vi "DataAnalysis.vi"() -> ()   [LabVIEW 2012]
doc: "DWTT主界面。\n\nname: 蒋松\nEmail：jiangsong@outlook.com"
uses:
  <vilib>/Utility/miscctls.llb/LVPoint32TypeDef.ctl
  <vilib>/Utility/miscctls.llb/LVRectTypeDef.ctl
panel:
  in  "FileExplore":string[](tree)
  in  "Exit":bool
  in  "Wave Select":u16(ring) items=["力/时间", "力/位移", "能量/位移", "位移/时间", "能量/时间", "速度/时间"]
  out "落锤高度":dbl
  out "MainXY":cluster{"Time":dbl[], "Energy":dbl[]}[](graph)
  out "冲击能量的特征值（J）":T1
  out "位移的特征值（mm）":T2
  out "环境温度":dbl
  out "材料名称":dbl
  out "系统状态":string="正常"
  out "落锤质量":dbl
  out "力的特征值（N）":T3
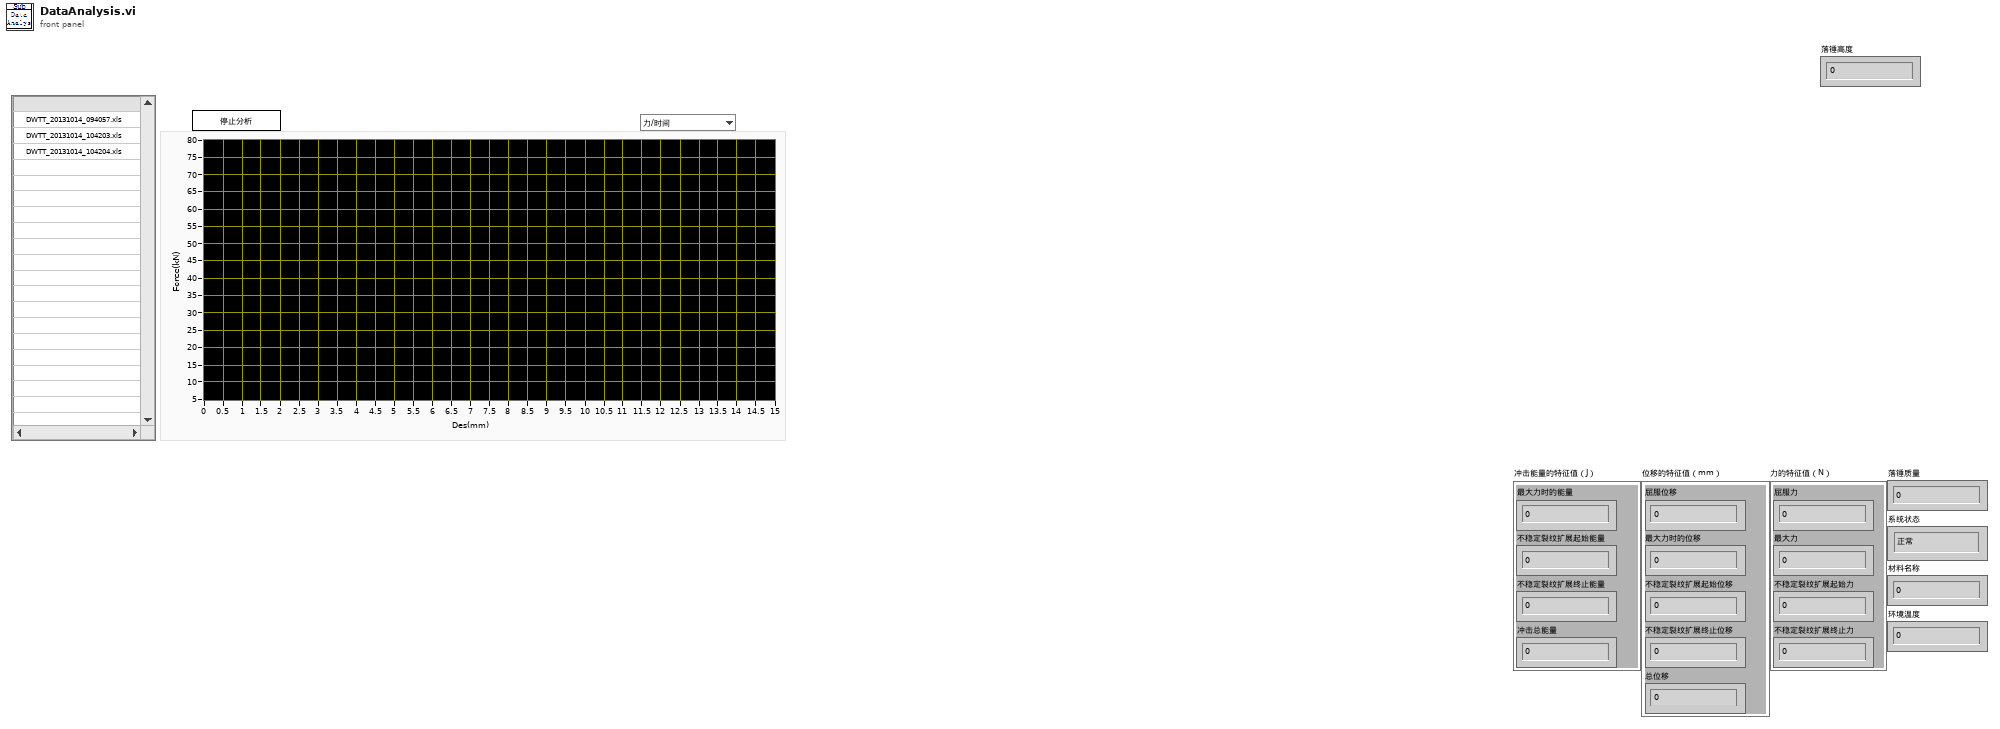
[diagram p1: front panel]
types:
  T1 = cluster{"最大力时的能量":dbl, "不稳定裂纹扩展起始能量":dbl, "不稳定裂纹扩展终止能量":dbl, "冲击总能量":dbl}
  T2 = cluster{"屈服位移":dbl, "最大力时的位移":dbl, "不稳定裂纹扩展起始位移":dbl, "不稳定裂纹扩展终止位移":dbl, "总位移":dbl}
  T3 = cluster{"屈服力":dbl, "最大力":dbl, "不稳定裂纹扩展起始力":dbl, "不稳定裂纹扩展终止力":dbl}
  T4 = enum32{"invalid app kind", "Development System", "Run Time System", "Student Edition", "Embedded LabVIEW", "Evaluation", "Custom"}
  T5 = cluster{"F/T":bool, "F/D":bool, "E/D":bool, "D/T":bool, "E/T":bool, "V/T":bool}
  T6 = typedef "LVRectTypeDef.ctl" = cluster{"Left":i16, "Top":i16, "Right":i16, "Bottom":i16}
  T7 = enum32{"Invalid", "Standard", "Closed", "Hidden", "Minimized", "Maximized"}
  T8 = cluster{"Core":cluster{"Current VI Reference":refnum<vi>, "Close Panel on Exit?":bool}, "EventPacket":cluster{"State":string, "data":variant}, "RawData":cluster{"Time":dbl[], "Force":dbl[], "Displacement":dbl[], "Velocity":dbl[], "Energy":dbl[]}[], "Tree Out":refnum<vi>, "XYData":cluster{"X":dbl[], "Y":dbl[]}[], "FilePathArray":path[], "FilePath":path, "MultiDataArray":cluster{"XYData":cluster{"X":dbl[], "Y":dbl[]}[]}[], "MultiPlot":cluster{"F/T":cluster{"X":dbl[], "Y":dbl[]}[], "F/D":cluster{"X":dbl[], "Y":dbl[]}[], "E/D":cluster{"X":dbl[], "Y":dbl[]}[], "D/T":cluster{"X":dbl[], "Y":dbl[]}[], "E/T":cluster{"X":dbl[], "Y":dbl[]}[], "V/T":cluster{"X":dbl[], "Y":dbl[]}[]}, "ChooseGraph":cluster{"F/T":bool, "F/D":bool, "E/D":bool, "D/T":bool, "E/T":bool, "V/T":bool}, "XYDataResult":cluster{"X":dbl[], "Y":dbl[]}[], "ScaleLabelText":cluster{"X":string, "Y":string}, "ScaleLable":cluster{"T":string, "F":string, "D":string, "E":string, "V":string}}
  T9 = cluster{"data name":string, "drag data":variant}[]
  T10 = typedef "LVPoint32TypeDef.ctl" = cluster{"Horizontal":i32, "Vertical":i32}
  T11 = cluster{"T":string, "F":string, "D":string, "E":string, "V":string}
  T12 = cluster{"F/T":cluster{"X":dbl[], "Y":dbl[]}[], "F/D":cluster{"X":dbl[], "Y":dbl[]}[], "E/D":cluster{"X":dbl[], "Y":dbl[]}[], "D/T":cluster{"X":dbl[], "Y":dbl[]}[], "E/T":cluster{"X":dbl[], "Y":dbl[]}[], "V/T":cluster{"X":dbl[], "Y":dbl[]}[]}
  T13 = cluster{"XYData":cluster{"X":dbl[], "Y":dbl[]}[]}[]
  T14 = cluster{"Time":dbl[], "Force":dbl[], "Displacement":dbl[], "Velocity":dbl[], "Energy":dbl[]}[]
  T15 = cluster{"Current VI Reference":refnum<vi>, "Close Panel on Exit?":bool}
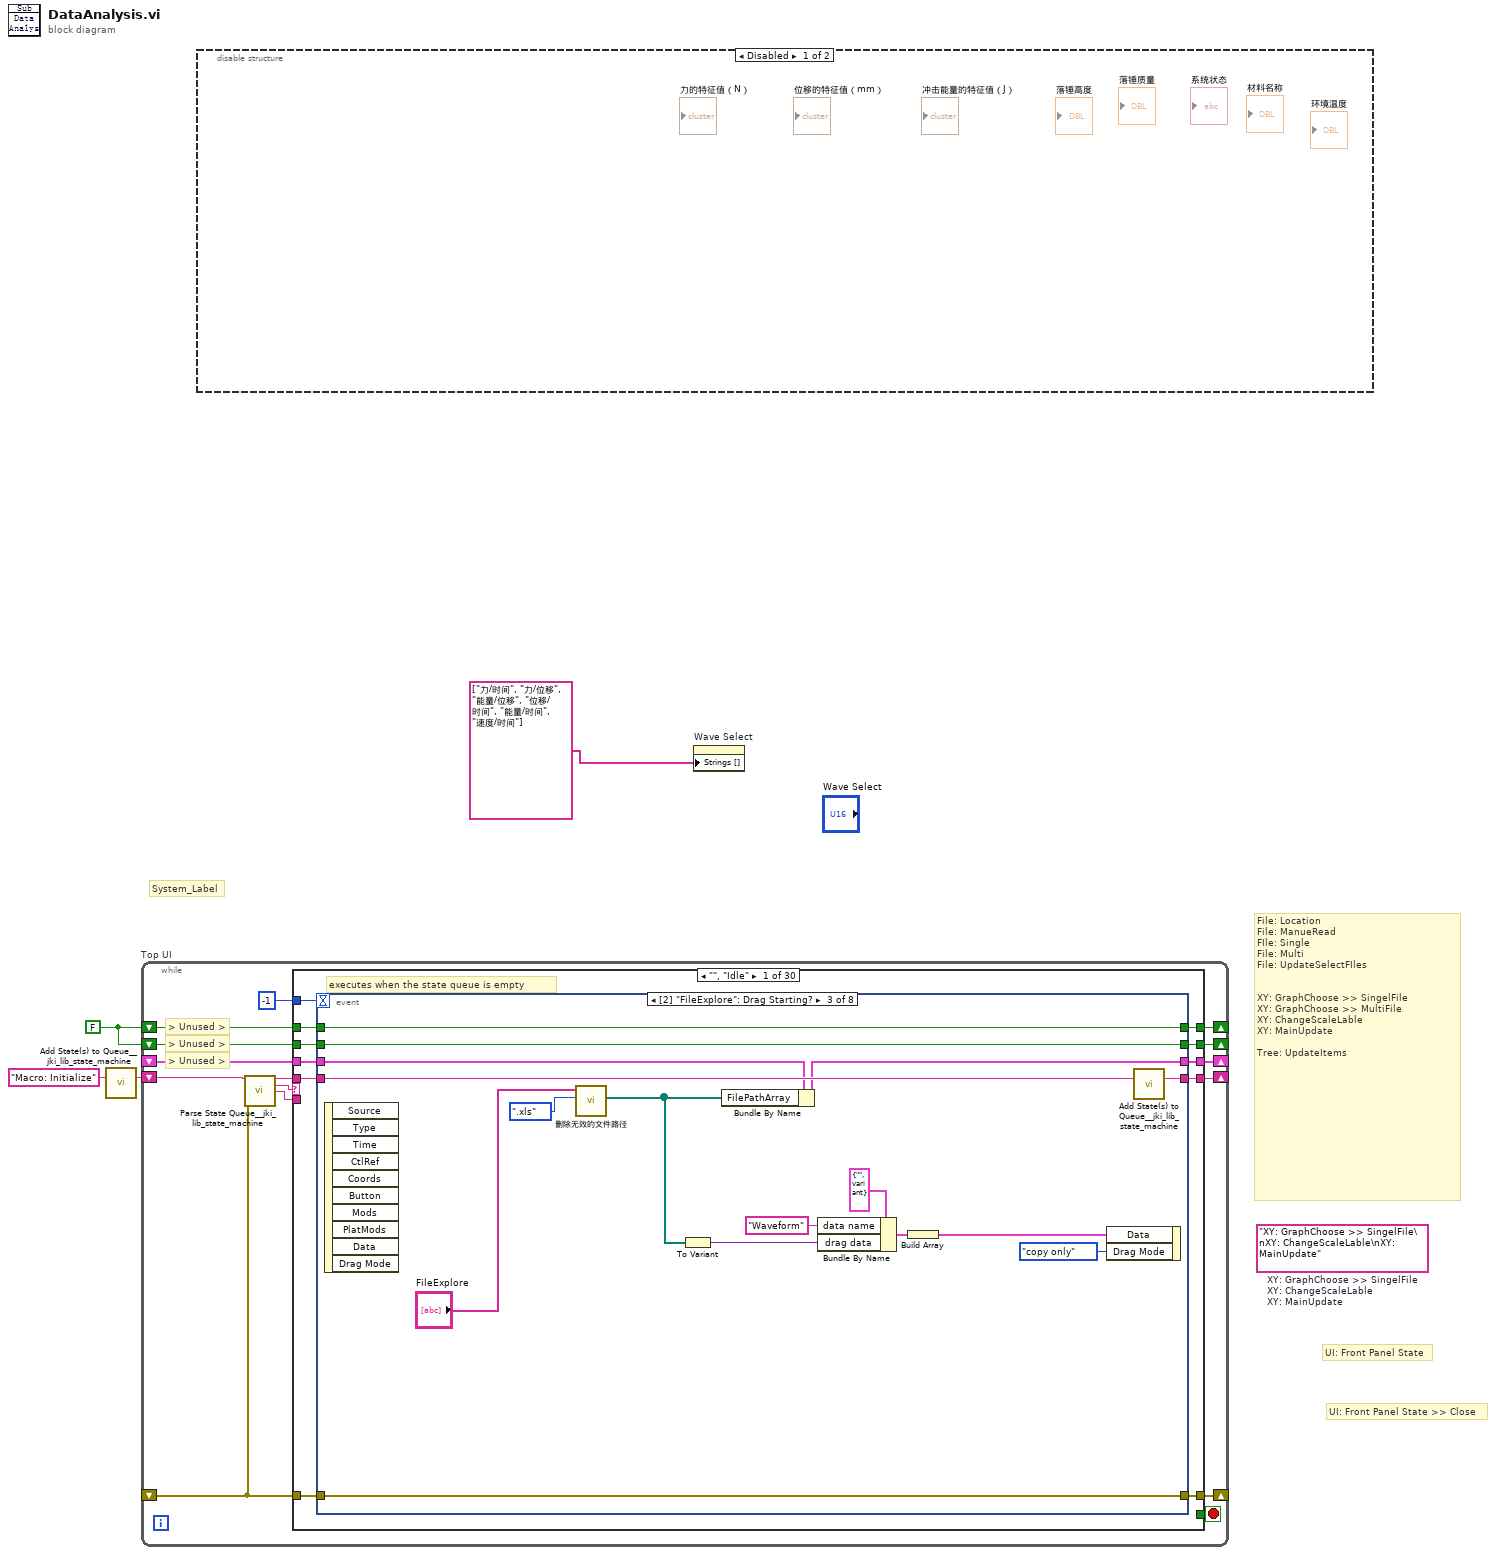
[diagram p0: block diagram]
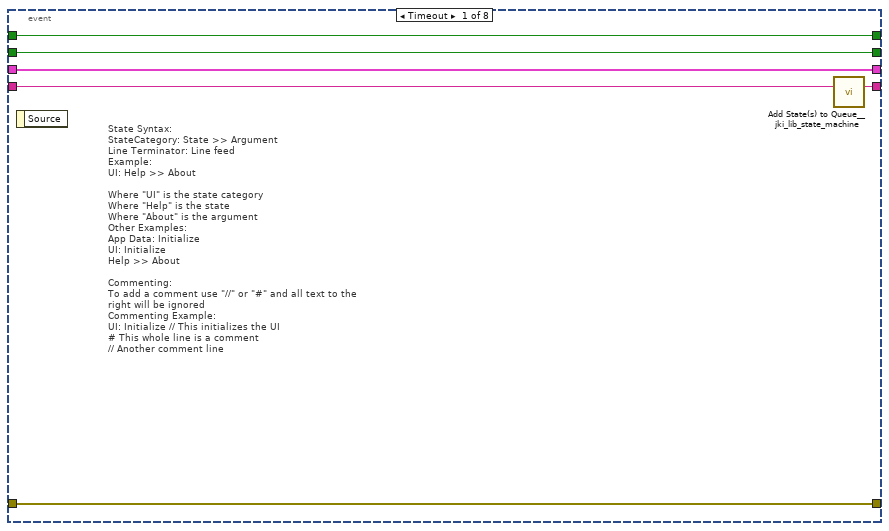
[diagram p3: hidden frame]
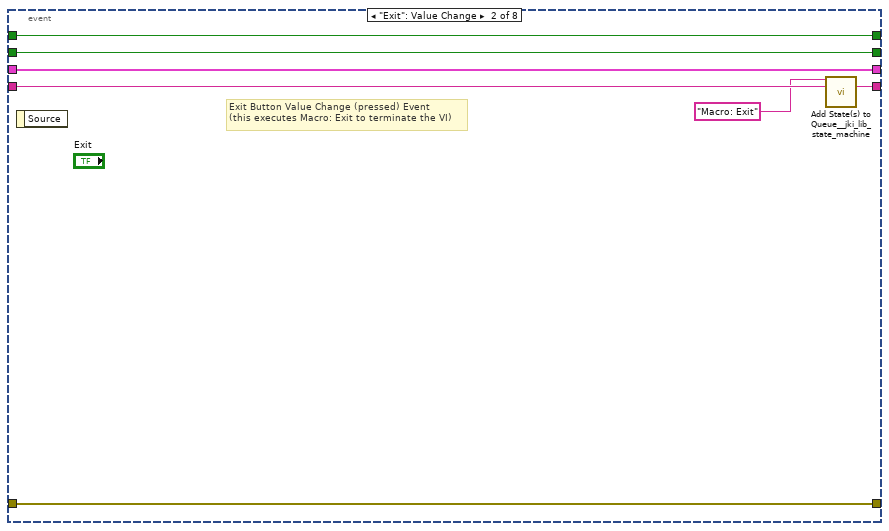
[diagram p4: hidden frame]
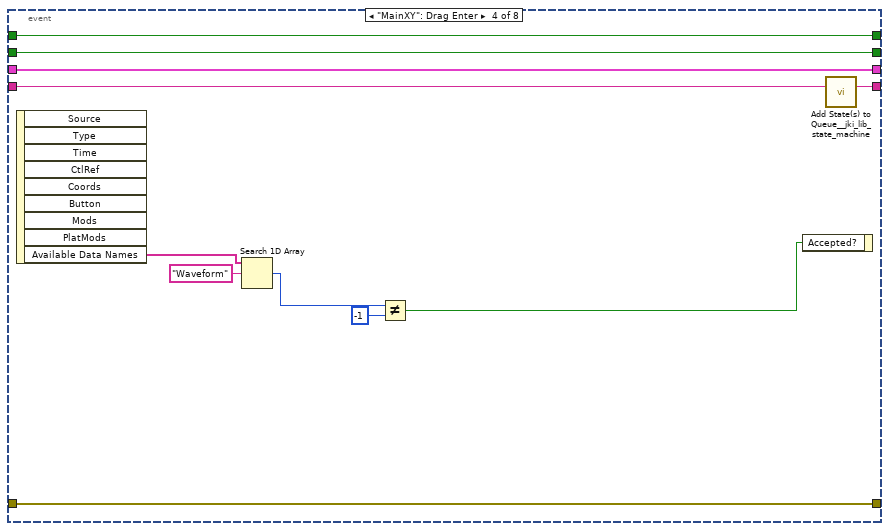
[diagram p5: hidden frame]
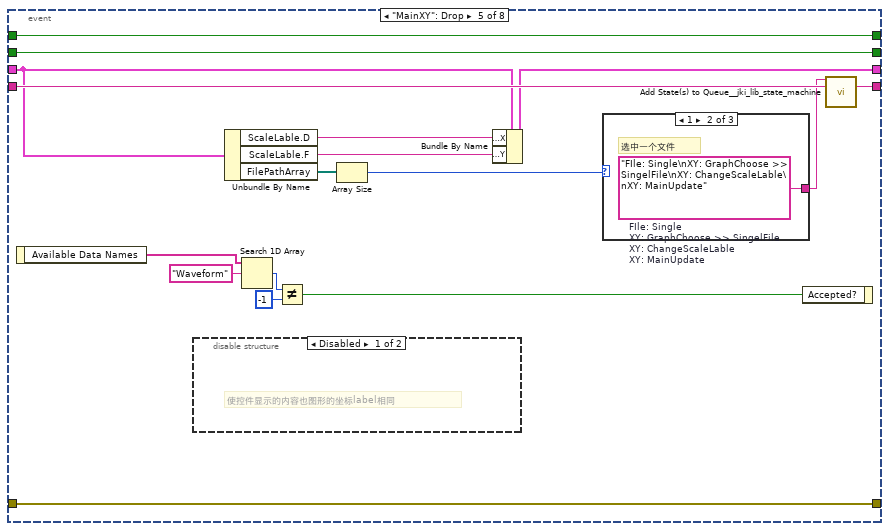
[diagram p6: hidden frame]
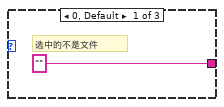
[diagram p8: hidden frame]
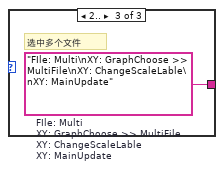
[diagram p9: hidden frame]
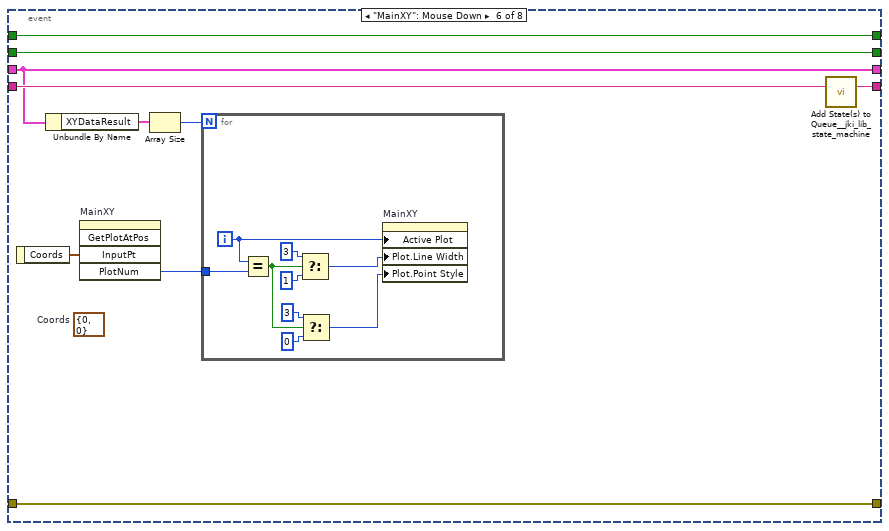
[diagram p10: hidden frame]
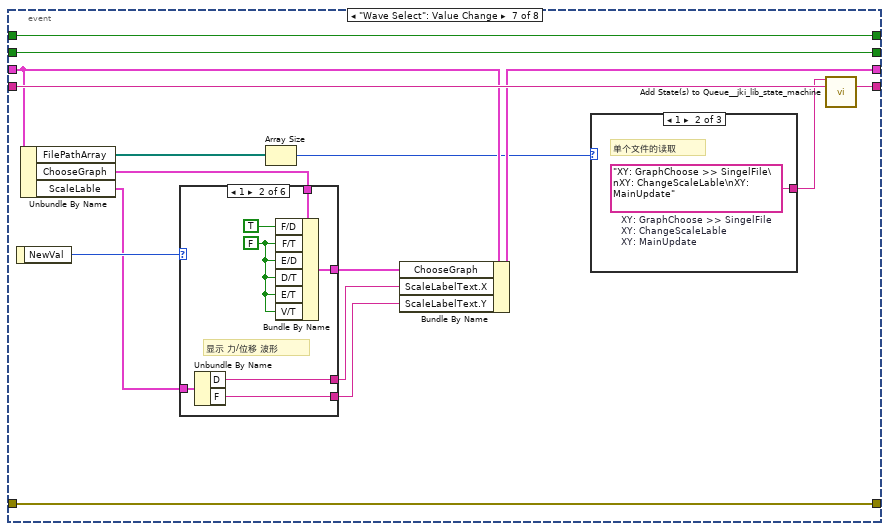
[diagram p11: hidden frame]
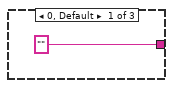
[diagram p12: hidden frame]
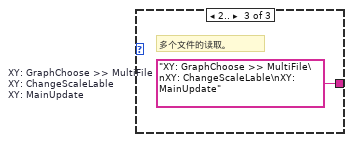
[diagram p13: hidden frame]
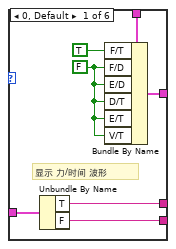
[diagram p14: hidden frame]
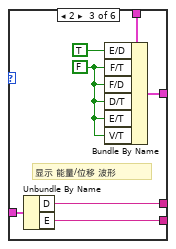
[diagram p15: hidden frame]
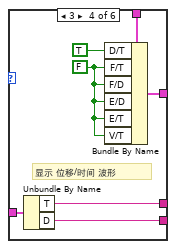
[diagram p16: hidden frame]
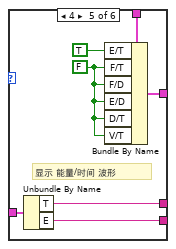
[diagram p17: hidden frame]
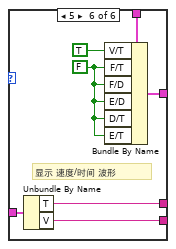
[diagram p18: hidden frame]
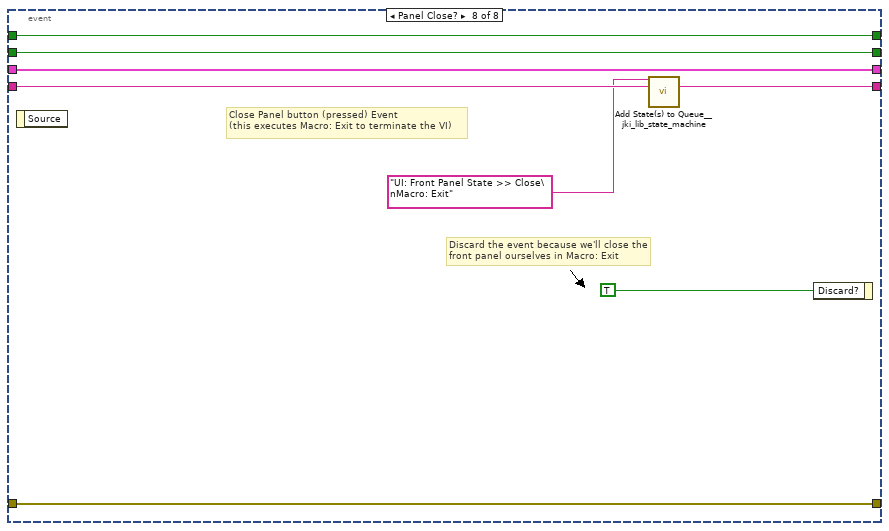
[diagram p19: hidden frame]
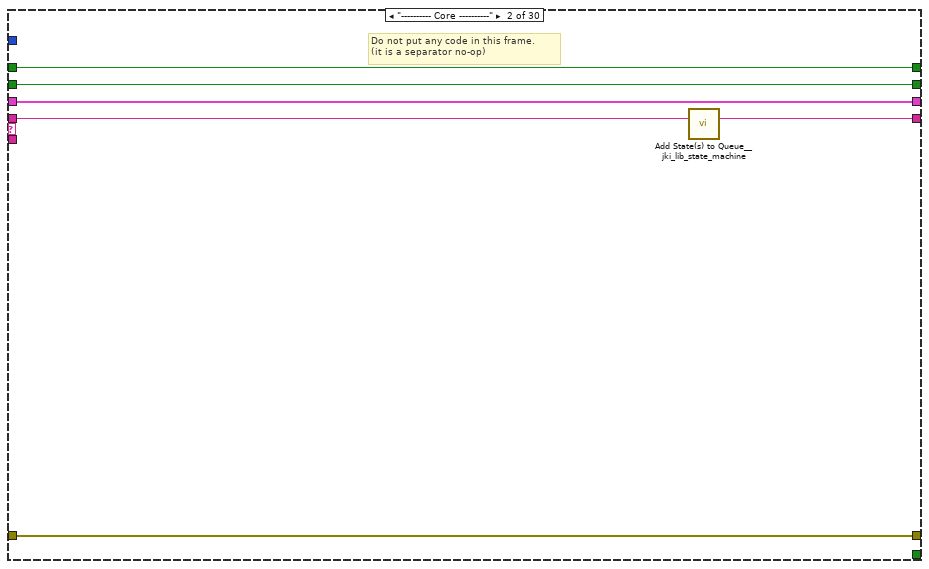
[diagram p20: hidden frame]
diagram:
  (unwired) "XY: GraphChoose >> SingelFile\nXY: ChangeScaleLable\nXY: MainUpdate"  # XY: GraphChoose >> SingelFile XY: ChangeScaleLable XY: MainUpdate
  w2 = FALSE
  # "UI: Front Panel State >> Close"
  # "UI: Front Panel State"
  # "File: Location\nFile: ManueRead\nFIle: Single\nFile: Multi\nFile: UpdateSelectFIles\n\n\nXY: GraphChoose >> SingelFile\nXY: GraphChoose >> MultiFile \nXY: ChangeScaleLable\nXY: MainUpdate\n\nTree: UpdateItems"
  # "System_Label"
  n1 = call "Add State(s) to Queue__jki_lib_state_machine.vi"("State(s) in (\"\")"="Macro: Initialize") -> ("States Out"=w3:string)  [unwired: 14 in]
  n2 = while "Top UI" {
    shift-right: [w12] -> _
    shift-left: _ -> [w11]
    shift-right: [w15] -> _
    shift-left: _ -> [w9]
    shift-right: [w14] -> _
    shift-left: w3 -> [w16]
    shift-right: [w7] -> _
    shift-left: w2 -> [w8]
    shift-right: [w5] -> _
    shift-left: w2 -> [w6]
    stop <- w13 stop-if-true
    # "> Unused >"
    # "> Unused >"
    # "> Unused >"
    n3 = call "Parse State Queue__jki_lib_state_machine.vi"("State Queue"=w16, "Error In (no error)"=w9) -> ("Remaining States"=w18:string, "Current State"=w19:string, "Arguments"=w17:string)  [unwired: 11 in]
    n4 = case shown="\"\", \"Idle\"" w19 {
      selector: w19 -> [_ _ w187 _ _ _ _ _ _ _ _ _ _ _ _ _ _ _ _ _ _ _ _ _ _ _ _ _ _ _]
      tunnel: w18 -> [w30 w184 w191 w211 w219 w226 w232 w251 w260 w266 w272 w282 w295 w323 w329 w336 w348 w354 w360 w374 w384 w397 w408 w414 w425 w444 w451 w457 w463 w469]
      tunnel: w17 -> [_ _ _ _ _ _ _ _ _ _ _ w277 w289 _ _ _ _ _ _ _ _ _ _ _ w420 _ _ _ _ _]
      tunnel: w11 -> [w28 w181 w189 w202 w216 w220 w229 _ w253 w263 w270 w280 w291 w320 w326 w333 w341 w351 w355 w367 w378 w386 w401 w409 w416 w439 w446 w454 w460 w466]
      tunnel: [w27 w182 w193 w208 errorcluster {"status"=FALSE, "code"=0, "source"=""} ("error out") w224 w230 w249 w256 w264 w269 w278 w292 w321 w327 w334 w346 w352 w358 w372 w382 w395 w406 w412 w423 w442 w449 w455 w461 w467] -> w15
      tunnel: w9 -> [w26 w182 w192 w208 w215 w224 w230 w249 w257 w264 w269 w279 w293 w321 w327 w334 w346 w352 w358 w372 w382 w395 w406 w412 w423 w442 w449 w455 w461 w467]
      tunnel: [w29 w183 w190 w210 w218 w225 w231 w250 w259 w265 w271 w281 w294 w322 w328 w335 w347 w353 w359 w373 w383 w396 w407 w413 w424 w443 w450 w456 w462 w468] -> w14
      tunnel: [_ _ _ _ _ TRUE _ _ _ _ _ _ _ _ _ _ _ _ _ _ _ _ _ _ _ _ _ _ _ _] -> w13
      tunnel: [w25 w181 w189 w209 w216 w220 w229 w247 w253 w263 w270 w280 w291 w320 w326 w333 w341 w351 w355 w366 w379 w385 w400 w409 w415 w439 w446 w454 w460 w466] -> w12
      tunnel: -1 ("Timeout") -> [w24 _ _ _ _ _ _ _ _ _ _ _ _ _ _ _ _ _ _ _ _ _ _ _ _ _ _ _ _ _]
      tunnel: w8 -> [w23 w179 w185 w198 w212 w221 w227 w246 w254 w261 w267 w275 w287 w318 w324 w330 w342 w349 w356 w370 w380 w393 w404 w410 w421 w440 w447 w452 w458 w464]
      tunnel: [w20 w179 w185 w198 w212 w221 w227 w246 w254 w261 w267 w275 w287 w318 w324 w330 w342 w349 w356 w370 w380 w393 w404 w410 w421 w440 w447 w452 w458 w464] -> w7
      tunnel: w6 -> [w22 w180 w186 w199 w213 w222 w228 w245 w255 w262 w268 w276 w288 w319 w325 w331 w343 w350 w357 w371 w381 w394 w405 w411 w422 w441 w448 w453 w459 w465]
      tunnel: [w21 w180 w186 w199 w213 w222 w228 w245 w255 w262 w268 w276 w288 w319 w325 w331 w343 w350 w357 w371 w381 w394 w405 w411 w422 w441 w448 w453 w459 w465] -> w5
      frame "", "Idle" {
        # "executes when the state queue is empty"
        n5 = event shown="[2] \"FileExplore\": Drag Starting?" {
          selector: _ -> [_ _ _ _ _ _ _ _]
          dyn-events: _ -> [_ _ _ _ _ _ _ _]
          timeout: w24 -> [_ _ _ _ _ _ _ _]
          tunnel: w30 -> [w36 w43 w59 w70 w87 w100 w125 w178]
          tunnel: [w35 w42 w58 w69 w86 w99 w124 w177] -> w29
          tunnel: w28 -> [w33 w37 w54 w65 w74 w94 w117 w175]
          tunnel: [w34 w41 w57 w68 w85 w98 w123 w176] -> w27
          tunnel: w26 -> [w34 w41 w57 w68 w85 w98 w123 w176]
          tunnel: [w33 w37 w53 w65 w73 w94 w116 w175] -> w25
          tunnel: w23 -> [w31 w38 w55 w66 w83 w96 w121 w171]
          tunnel: w22 -> [w32 w39 w56 w67 w84 w97 w122 w172]
          tunnel: [w32 w39 w56 w67 w84 w97 w122 w172] -> w21
          tunnel: [w31 w38 w55 w66 w83 w96 w121 w171] -> w20
          event Timeout {
            # "State Syntax:\nStateCategory: State >> Argument\nLine Terminator: Line feed\nExample:\nUI: Help >> About\n\nWhere \"UI\" is the state category\nWhere \"Help\" is the state\nWhere \"About\" is the argument\nOther Examples:\nApp Data: Initialize\nUI: Initialize\nHelp >> About\n\nCommenting:\nTo add a comment use \"//\" or \"#\" and all text to the right will be ignored\nCommenting Example:\nUI: Initialize // This initializes the UI\n# This whole line is a comment\n// Another comment line"
            n6 = event-data() -> ()  [unwired: 1 in, 1 out]
            n7 = call "Add State(s) to Queue__jki_lib_state_machine.vi"("State(s) in (\"\")"=w36) -> ("States Out"=w35:string)  [unwired: 14 in]
          }
          event "Exit": Value Change {
            # "Exit Button Value Change (pressed) Event\n(this executes Macro: Exit to terminate the VI)"
            n8 = event-data() -> ()  [unwired: 1 in, 1 out]
            n9 = call "Add State(s) to Queue__jki_lib_state_machine.vi"("State(s) in Front (\"\")"="Macro: Exit", "State(s) in (\"\")"=w43) -> ("States Out"=w42:string)  [unwired: 13 in]
          }
          event "FileExplore": Drag Starting? {
            n10 = event-data() -> ()  [unwired: 1 in, 10 out]
            n11 = call "删除无效的文件路径.vi"("Enum"=enum16{".xls", ".txt"}.".xls", "NewVal"="FileExplore") -> ("FilePathArray"=w45:path[])  [unwired: 7 in, 2 out]
            n12 = To Variant(anything=w45) -> (Variant=w44:variant)
            n13 = Bundle By Name(cluster=w54, "FilePathArray"=w45) -> (w53:T8)
            n14 = Bundle By Name(cluster=cluster{"data name":string, "drag data":variant} {"data name"="", "drag data"=variant}, "data name"="Waveform", "drag data"=w44) -> (w48:cluster{"data name":string, "drag data":variant})
            n15 = Build Array(w48) -> (w47:T9)
            n16 = event-data("Data"=w47, "Drag Mode"=enum32{"copy or move", "copy only", "move only"}."copy only") -> ()  [unwired: 1 in, 1 out]
            n17 = call "Add State(s) to Queue__jki_lib_state_machine.vi"("State(s) in (\"\")"=w59) -> ("States Out"=w58:string)  [unwired: 14 in]
          }
          event "MainXY": Drag Enter {
            n18 = event-data() -> ("Available Data Names"=w64:string[])  [unwired: 1 in, 8 out]
            n19 = Search 1D Array(1D array=w64, element="Waveform") -> (index of element=w62:i32)  [unwired: 1 in]
            n20 = Not Equal?(x=w62, y=-1) -> (x != y?=w60:bool)
            n21 = event-data("Accepted?"=w60) -> ()  [unwired: 1 in, 1 out]
            n22 = call "Add State(s) to Queue__jki_lib_state_machine.vi"("State(s) in (\"\")"=w70) -> ("States Out"=w69:string)  [unwired: 14 in]
          }
          event "MainXY": Drop {
            n23 = event-data() -> ("Available Data Names"=w82:string[])  [unwired: 1 in]
            n24 = disable-structure shown="Disabled" {
              frame Disabled {
                # "使控件显示的内容也图形的坐标label相同"
              }
              frame Enabled {
              }
            }
            n25 = Unbundle By Name(w74) -> ("ScaleLable.D"=w72:string, "ScaleLable.F"=w71:string, "FilePathArray"=w76:path[])
            n26 = Search 1D Array(1D array=w82, element="Waveform") -> (index of element=w80:i32)  [unwired: 1 in]
            n27 = Not Equal?(x=w80, y=-1) -> (x != y?=w78:bool)
            n28 = Array Size(array=w76) -> (size(s)=w75:i32)
            n29 = Bundle By Name(cluster=w74, "ScaleLabelText.X"=w72, "ScaleLabelText.Y"=w71) -> (w73:T8)
            n30 = case shown="1" w75 {
              tunnel: ["" w89 w90] -> w77
              frame 0, Default {
                # "选中的不是文件"
              }
              frame 1 {
                w89 = "FIle: Single\nXY: GraphChoose >> SingelFile\nXY: ChangeScaleLable\nXY: MainUpdate"  # FIle: Single XY: GraphChoose >> SingelFile XY: ChangeScaleLable XY: MainUpdate
                # "选中一个文件"
              }
              frame 2.. {
                w90 = "FIle: Multi\nXY: GraphChoose >> MultiFile\nXY: ChangeScaleLable\nXY: MainUpdate"  # FIle: Multi XY: GraphChoose >> MultiFile XY: ChangeScaleLable XY: MainUpdate
                # "选中多个文件"
              }
            }
            n31 = event-data("Accepted?"=w78) -> ()  [unwired: 1 in, 1 out]
            n32 = call "Add State(s) to Queue__jki_lib_state_machine.vi"("State(s) in Front (\"\")"=w77, "State(s) in (\"\")"=w87) -> ("States Out"=w86:string)  [unwired: 13 in]
          }
          event "MainXY": Mouse Down {
            (unwired) T10 {"Horizontal"=0, "Vertical"=0}  # Coords
            n33 = event-data() -> ("Coords"=w95:T10)  [unwired: 1 in]
            n34 = Unbundle By Name(w94) -> ("XYDataResult"=w93:cluster{"X":dbl[], "Y":dbl[]}[])
            n35 = invoke on="MainXY" class="XYGraph (strict)" method="GetPlotAtPos"("InputPt"=w95) -> ("PlotNum"=w91:i32)  [unwired: 4 in, 4 out]
            n36 = Array Size(array=w93) -> (size(s)=w92:i32)
            n37 = for {
              N: w92 -> [_]
              tunnel: w91 -> [w108]
              i -> [w109]
              n38 = Equal?(x=w109, y=w108) -> (x = y?=w102:bool)
              n39 = Select(t=u8 3, s=w102, f=u8 1) -> (s? t:f=w105:u8)
              n40 = Select(t=u8 3, s=w102, f=u8 0) -> (s? t:f=w101:u8)
              n41 = property on="MainXY" class="XYGraph (strict)"("Active Plot"=w109, "Plot.Line Width"=w105, "Plot.Point Style"=w101) -> ()  [unwired: 2 in, 2 out]
            }
            n42 = call "Add State(s) to Queue__jki_lib_state_machine.vi"("State(s) in (\"\")"=w100) -> ("States Out"=w99:string)  [unwired: 14 in]
          }
          event "Wave Select": Value Change {
            n43 = event-data() -> ("NewVal"=w120:u16)  [unwired: 1 in]
            n44 = Unbundle By Name(w117) -> ("FilePathArray"=w114:path[], "ChooseGraph"=w119:T5, "ScaleLable"=w112:T11)
            n45 = case shown="1" w120 {
              tunnel: w119 -> [w134 w141 w148 w155 w162 w169]
              tunnel: [w133 w140 w147 w154 w161 w168] -> w118
              tunnel: w112 -> [w131 w138 w145 w152 w159 w166]
              tunnel: [w130 w137 w144 w151 w158 w165] -> w111
              tunnel: [w129 w136 w143 w150 w157 w164] -> w110
              frame 0, Default {
                w135 = FALSE
                # "显示 力/时间 波形"
                n46 = Unbundle By Name(w131) -> ("T"=w130:string, "F"=w129:string)
                n47 = Bundle By Name(cluster=w134, "F/T"=TRUE, "F/D"=w135, "E/D"=w135, "D/T"=w135, "E/T"=w135, "V/T"=w135) -> (w133:T5)
              }
              frame 1 {
                w142 = FALSE
                # "显示 力/位移 波形"
                n48 = Unbundle By Name(w138) -> ("D"=w137:string, "F"=w136:string)
                n49 = Bundle By Name(cluster=w141, "F/D"=TRUE ("F/T"), "F/T"=w142, "E/D"=w142, "D/T"=w142, "E/T"=w142, "V/T"=w142) -> (w140:T5)
              }
              frame 2 {
                w149 = FALSE
                # "显示 能量/位移 波形"
                n50 = Unbundle By Name(w145) -> ("D"=w144:string, "E"=w143:string)
                n51 = Bundle By Name(cluster=w148, "E/D"=TRUE ("F/T"), "F/T"=w149, "F/D"=w149, "D/T"=w149, "E/T"=w149, "V/T"=w149) -> (w147:T5)
              }
              frame 3 {
                w156 = FALSE
                # "显示 位移/时间 波形"
                n52 = Unbundle By Name(w152) -> ("T"=w151:string, "D"=w150:string)
                n53 = Bundle By Name(cluster=w155, "D/T"=TRUE ("F/T"), "F/T"=w156, "F/D"=w156, "E/D"=w156, "E/T"=w156, "V/T"=w156) -> (w154:T5)
              }
              frame 4 {
                w163 = FALSE
                # "显示 能量/时间 波形"
                n54 = Unbundle By Name(w159) -> ("T"=w158:string, "E"=w157:string)
                n55 = Bundle By Name(cluster=w162, "E/T"=TRUE ("F/T"), "F/T"=w163, "F/D"=w163, "E/D"=w163, "D/T"=w163, "V/T"=w163) -> (w161:T5)
              }
              frame 5 {
                w170 = FALSE
                # "显示 速度/时间 波形"
                n56 = Unbundle By Name(w166) -> ("T"=w165:string, "V"=w164:string)
                n57 = Bundle By Name(cluster=w169, "V/T"=TRUE ("F/T"), "F/T"=w170, "F/D"=w170, "E/D"=w170, "D/T"=w170, "E/T"=w170) -> (w168:T5)
              }
            }
            n58 = Array Size(array=w114) -> (size(s)=w113:i32)
            n59 = Bundle By Name(cluster=w117, "ChooseGraph"=w118, "ScaleLabelText.X"=w111, "ScaleLabelText.Y"=w110) -> (w116:T8)
            n60 = case shown="1" w113 {
              tunnel: ["" w127 w128] -> w115
              frame 0, Default {
              }
              frame 1 {
                w127 = "XY: GraphChoose >> SingelFile\nXY: ChangeScaleLable\nXY: MainUpdate"  # XY: GraphChoose >> SingelFile XY: ChangeScaleLable XY: MainUpdate
                # "单个文件的读取"
              }
              frame 2.. {
                w128 = "XY: GraphChoose >> MultiFile\nXY: ChangeScaleLable\nXY: MainUpdate"  # XY: GraphChoose >> MultiFile XY: ChangeScaleLable XY: MainUpdate
                # "多个文件的读取。"
              }
            }
            n61 = call "Add State(s) to Queue__jki_lib_state_machine.vi"("State(s) in Front (\"\")"=w115, "State(s) in (\"\")"=w125) -> ("States Out"=w124:string)  [unwired: 13 in]
          }
          event Panel Close? {
            # "Discard the event because we'll close the front panel ourselves in Macro: Exit"
            # "Close Panel button (pressed) Event\n(this executes Macro: Exit to terminate the VI)"
            n62 = event-data() -> ()  [unwired: 1 in, 1 out]
            n63 = call "Add State(s) to Queue__jki_lib_state_machine.vi"("State(s) in Front (\"\")"="UI: Front Panel State >> Close\nMacro: Exit", "State(s) in (\"\")"=w178) -> ("States Out"=w177:string)  [unwired: 13 in]
            n64 = event-data("Discard?"=TRUE) -> ()  [unwired: 1 in, 1 out]
          }
        }
      }
      frame "---------- Core ----------" {
        # "Do not put any code in this frame.\n(it is a separator no-op)"
        n65 = call "Add State(s) to Queue__jki_lib_state_machine.vi"("State(s) in (\"\")"=w184) -> ("States Out"=w183:string)  [unwired: 14 in]
      }
      frame Default {
        w196 = 42 items=["No error", "Argument error", "Memory is full", "Out of zone", "End of file", "File already open", "Generic file I/O error", "File not found", "File permission error", "Disk is full", "Duplicate path", "Too many files open", "System feature not enabled", "Resource file not found", "Cannot add resource", "Resource not found", "Image not found", "Image memory error", "Pen does not exist", "Config type invalid", "Config token not found", "Config parse error", "Config memory error", "Bad external code format", "Bad external code offset", "External code not present", "Null window", "Destroy window error", "Null menu", "Print aborted", "Bad print record", "Print driver error", "Windows error during printing", "Memory error during printing", "Print dialog error", "Generic print error", "Invalid device refnum", "Device not found", "Device parameter error", "Device unit error", "Cannot open device", "Device call aborted", "Generic error", "Cancelled by user", "Object ID too low", "Object ID too high", "Object not in heap", "Unknown heap", "Unknown object (invalid DefProc)", "Unknown object (DefProc not in table)", "Message out of range", "Invalid (null) method", "Unknown message", "Manager call not supported", "Bad address", "Network operation in progress", "Network operation timed out", "Connection is busy", "Network attribute not supported", "Network error", "Address in use", "System out of memory", "Connection aborted", "Connection refused", "Not connected", "Already connected", "Connection closed", "Initialization error (interapplication manager)", "Bad occurrence", "Wait on unbound occurrence handler", "Occurrence queue overflow", "Datalog type conflict", "Unused", "Unrecognized type (interapplication manager)", "Memory corrupt", "Failed to make temporary DLL", "Old CIN version", "Drag socket not found", "Failed to load drop-object", "Failed to register OLE object", "Failed to release OLE object", "Format specifier type mismatch", "Unknown format specifier", "Too few format specifiers", "Too many format specifiers", "Scan failed", "Newer CIN version", "Error converting to variant", "Runtime menu error", "Password tampered", "Variant attribute not found", "Incompatible variant data type", "Event data is not available", "Event Store is not present", "Occurrence is not found", "Event Queue is not created", "Event info is not available", "Refnum passed is NULL", "Error retrieving Class GUID", "Error retrieving CoClass GUID", "Error retrieving TypeLib GUID.", "Bad built application magic bytes.", "Specific driver is different from the specific driver associated with the Logical Name.", "There is no session opened to the class driver.", "Max Error", "MAX - Error with config objects", "MAX - Error loading configuration", "MAX - Group not supported"]
        # "Current State"
        # "Do not delete, rename, or modify this frame.\n(this is used to capture unhandled states and typos)"
        # "Handle mistyped state name (developer tool)"
        n66 = Format Into String(format string="Software Exception: Unhandled State \"%s\"." ("message"), error in=w192, w187) -> (resulting string=w195:string, error out=w194:errorcluster)  [unwired: 1 in]
        n67 = call <vilib>:"Error Cluster From Error Code.vi"("show call chain? (False)"=TRUE, "error in (no error)"=w194, "error message (\"\")"=w195, "error code (0)"=w196) -> ("error out"=w193:errorcluster)  [unwired: 5 in]
        n68 = call "Add State(s) to Queue__jki_lib_state_machine.vi"("State(s) in (\"\")"=w191) -> ("States Out"=w190:string)  [unwired: 14 in]
      }
      frame "Initialize Core Data" {
        # "Do not delete, rename, or modify this frame.\n(this is used to determine panel behavior on exit)"
        # "originally closed?"
        # "exe?"
        # "If panel starts closed or is an EXE, then close it when we exit"
        n69 = property class="VI"() -> ("Front Panel.Open"=w207:bool)  [unwired: 2 in, 2 out]
        n70 = property class="App"() -> ("App.Kind"=w206:T4)  [unwired: 2 in, 2 out]
        n71 = control-ref of="Current VI Reference"() -> (w200:refnum<vi>)
        n72 = Not(x=w207) -> (.not. x?=w204:bool)
        n73 = Equal?(x=w206, y=T4."Run Time System" ("Application:Kind")) -> (x = y?=w203:bool)
        n74 = Or(x=w204, y=w203) -> (x .or. y?=w201:bool)
        n75 = Bundle By Name(cluster=w202, "Core.Current VI Reference"=w200, "Core.Close Panel on Exit?"=w201) -> (w209:T8)
        n76 = call "Add State(s) to Queue__jki_lib_state_machine.vi"("State(s) in (\"\")"=w211) -> ("States Out"=w210:string)  [unwired: 14 in]
      }
      frame "Error Handler" {
        # "Unhandled Error -- Display it"
        # "Handle any errors here.\nYou can also output any states to clean-up after errors occur"
        # "Clear error"
        n77 = call <vilib>:"General Error Handler.vi"("error in (no error)"=w215) -> ()  [unwired: 10 in, 5 out]
        n78 = call "Add State(s) to Queue__jki_lib_state_machine.vi"("State(s) in Front (\"\")"="/* Post Error States", "State(s) in (\"\")"=w219) -> ("States Out"=w218:string)  [unwired: 13 in]
      }
      frame "Exit" {
        # "Do not put any code in this frame.\n(No errors that occur here will be handled.)"
        n79 = call "Add State(s) to Queue__jki_lib_state_machine.vi"("State(s) in (\"\")"=w226) -> ("States Out"=w225:string)  [unwired: 14 in]
      }
      frame "---------- Data ----------" {
        # "Do not put any code in this frame.\n(It is a separator no-op. You can make a copy of this frame to create a new Data frame)"
        n80 = call "Add State(s) to Queue__jki_lib_state_machine.vi"("State(s) in (\"\")"=w232) -> ("States Out"=w231:string)  [unwired: 14 in]
      }
      frame "Data: Initialize" {
        w233 = T11 {"T"="T(ms)", "F"="Force(kN)", "D"="Des(mm)", "E"="E(kJ)", "V"="V(m1s)"}  # ScaleLable
        w234 = cluster{"X":string, "Y":string} {"X"="", "Y"=""}  # ScaleLabelText
        w236 = T5 {"F/T"=FALSE, "F/D"=TRUE, "E/D"=FALSE, "D/T"=FALSE, "E/T"=FALSE, "V/T"=FALSE}  # ChooseGraph
        w235 = cluster{"X":dbl[], "Y":dbl[]}[] []  # XYDataResult
        w237 = T12 {"F/T"=[], "F/D"=[], "E/D"=[], "D/T"=[], "E/T"=[], "V/T"=[]}  # MultiPlot
        w238 = T13 []  # MultiDataArray
        w239 = cluster{"X":dbl[], "Y":dbl[]}[] []  # XYData
        w240 = path ""  # FilePath
        w241 = path[] []  # FilePathArray
        w243 = T14 []  # RawData
        w248 = T15 {"Current VI Reference"=refnum, "Close Panel on Exit?"=FALSE}  # Core
        # "Initialize the shift-register data, here.\n(data names are defined by what you wire into the bundle function)"
        n81 = Bundle("Core"=w248, "EventPacket"=cluster{"State":string, "data":variant} {"State"="", "data"=variant}, "RawData"=w243, "Tree Out"=refnum<vi> refnum, "XYData"=w239, "FilePathArray"=w241, "FilePath"=w240, "MultiDataArray"=w238, "MultiPlot"=w237, "ChooseGraph"=w236, "XYDataResult"=w235, "ScaleLabelText"=w234, "ScaleLable"=w233) -> (w247:T8)  [unwired: 1 in]
        n82 = call "Add State(s) to Queue__jki_lib_state_machine.vi"("State(s) in (\"\")"=w251) -> ("States Out"=w250:string)  [unwired: 14 in]
      }
      frame "Data: Cleanup" {
        # "Cleanup any data and references, here.\n(this is called automatically, by the Macro: Exit)"
        n83 = Unbundle By Name(w253) -> ("Core.Current VI Reference"=w258:refnum<vi>)
        n84 = Close Reference(reference=w258, error in (no error)=w257) -> (error out=w256:errorcluster)
        n85 = Bundle By Name(cluster=w253, "ChooseGraph"=T5 {"F/T"=FALSE, "F/D"=TRUE, "E/D"=FALSE, "D/T"=FALSE, "E/T"=FALSE, "V/T"=FALSE}) -> ()  [unwired: 1 out]
        n86 = call "Add State(s) to Queue__jki_lib_state_machine.vi"("State(s) in (\"\")"=w260) -> ("States Out"=w259:string)  [unwired: 14 in]
      }
      frame "---------- UI ----------" {
        # "Do not put any code in this frame.\n(It is a separator no-op. You can make a copy of this frame to create a new UI frame)"
        n87 = call "Add State(s) to Queue__jki_lib_state_machine.vi"("State(s) in (\"\")"=w266) -> ("States Out"=w265:string)  [unwired: 14 in]
      }
      frame "UI: Initialize" {
        # "Initialize the User Interface, here.\n(this is called automatically, by the Macro: Init)"
        n88 = invoke on="MainXY" class="XYGraph (strict)" method="Reinit To Default"() -> ()  [unwired: 3 in, 3 out]
        n89 = call "Add State(s) to Queue__jki_lib_state_machine.vi"("State(s) in (\"\")"=w272) -> ("States Out"=w271:string)  [unwired: 14 in]
        n90 = disable-structure shown="Enabled" {
          frame Disabled {
            n91 = control-ref of="This VI"() -> (w274:refnum<vi>)
            n92 = property class="VI"(reference=w274, "Front Panel.PanelBounds"=T6 {"Left"=0, "Top"=0, "Right"=1280, "Bottom"=986} ("Front Panel Window:Panel Bounds")) -> ()  [unwired: 1 in, 2 out]
          }
          frame Enabled {
          }
        }
      }
      frame "UI: Cursor Set" {
        # "Argument"
        # "Set and Unset Cursor Busy.\n(Usage: \"UI: Cursor Set >> Busy|Idle\")"
        n93 = case shown="\"Idle\", Default" w277 {
          tunnel: w279 -> [w284 w286]
          tunnel: [w283 w285] -> w278
          frame "Idle", Default {
            n94 = call <vilib>:"Unset Busy.vi"("error in (no error)"=w284) -> ("error out"=w283:errorcluster)  [unwired: 10 in]
          }
          frame "Busy" {
            n95 = call <vilib>:"Set Busy.vi"("error in (no error)"=w286) -> ("error out"=w285:errorcluster)  [unwired: 9 in, 1 out]
          }
        }
        n96 = call "Add State(s) to Queue__jki_lib_state_machine.vi"("State(s) in (\"\")"=w282) -> ("States Out"=w281:string)  [unwired: 14 in]
      }
      frame "UI: Front Panel State" {
        # "Argument"
        # "Set Front Panel Open or Closed\n(Usage: \"UI: Front Panel State >> Open|Close\")"
        n97 = Unbundle By Name(w291) -> ("Core.Current VI Reference"=w290:refnum<vi>)
        n98 = case shown="\"Close\"" w289 {
          tunnel: w293 -> [w299 w312]
          tunnel: [w301 w313] -> w292
          tunnel: w290 -> [w300 w310]
          frame "Open", Default {
            n99 = property class="VI"(reference=w300, error in=w299) -> (reference out=w297:refnum<vi>, error out=w298:errorcluster, "Front Panel.Open"=w296:bool)
            n100 = case shown="True" w296 {
              tunnel: [w304 w307] -> w301
              tunnel: w298 -> [w303 w307]
              tunnel: w297 -> [w302 _]
              frame False {
                n101 = invoke class="VI" method="FP.Open"(reference=w302, error in=w303, "Activate"=TRUE, "State"=T7."Standard") -> (error out=w304:errorcluster)  [unwired: 1 in, 4 out]
              }
              frame True {
              }
            }
          }
          frame "Close" {
            n102 = property class="VI"(reference=w310, error in=w312) -> (reference out=w309:refnum<vi>, error out=w311:errorcluster, "Front Panel.Open"=w308:bool)
            n103 = case shown="True" w308 {
              tunnel: [w314 w317] -> w313
              tunnel: w311 -> [w314 w316]
              tunnel: w309 -> [_ w315]
              frame False {
              }
              frame True {
                n104 = invoke class="VI" method="FP.Close"(reference=w315, error in=w316) -> (error out=w317:errorcluster)  [unwired: 1 in, 2 out]
              }
            }
          }
        }
        n105 = call "Add State(s) to Queue__jki_lib_state_machine.vi"("State(s) in (\"\")"=w295) -> ("States Out"=w294:string)  [unwired: 14 in]
      }
      frame "UI: Controls" {
        # "Do not put any code in this frame.\n(It is a separator no-op. You can make a copy of this frame to create a new UI frame)"
        n106 = call "Add State(s) to Queue__jki_lib_state_machine.vi"("State(s) in (\"\")"=w323) -> ("States Out"=w322:string)  [unwired: 14 in]
      }
      frame "---------- Macro ----------" {
        # "Do not put any code in this frame.\n(It is a separator no-op. You can make a copy of this frame to create a new Macro frame)"
        n107 = call "Add State(s) to Queue__jki_lib_state_machine.vi"("State(s) in (\"\")"=w329) -> ("States Out"=w328:string)  [unwired: 14 in]
      }
      frame "Macro: Initialize" {
        # "Initialization Macro\n(This is called once, when the VI starts)"
        n108 = call "Add State(s) to Queue__jki_lib_state_machine.vi"("State(s) in Front (\"\")"="Data: Initialize\nInitialize Core Data\nUI: Initialize\nUI: Front Panel State >> Open\nFile: Location", "State(s) in (\"\")"=w336) -> ("States Out"=w335:string)  [unwired: 13 in]
      }
      frame "Macro: Exit" {
        # "Exit Macro\n(This is called once, when the VI exits)"
        n109 = Unbundle By Name(w341) -> ("Core.Close Panel on Exit?"=w345:bool)
        n110 = Select(t="UI: Front Panel State >> Close", s=w345, f="") -> (s? t:f=w338:string)
        n111 = call "Add State(s) to Queue__jki_lib_state_machine.vi"("State(s) in (\"\")"=w338, "State(s) at Back (\"\")"="Data: Cleanup\nExit") -> ("States Out"=w344:string)  [unwired: 13 in]
        n112 = call "Add State(s) to Queue__jki_lib_state_machine.vi"("State(s) in Front (\"\")"=w344, "State(s) in (\"\")"=w348) -> ("States Out"=w347:string)  [unwired: 13 in]
      }
      frame "----------- DAQ -----------" {
        n113 = call "Add State(s) to Queue__jki_lib_state_machine.vi"("State(s) in (\"\")"=w354) -> ("States Out"=w353:string)  [unwired: 14 in]
      }
      frame "------------File ------------" {
        n114 = call "Add State(s) to Queue__jki_lib_state_machine.vi"("State(s) in (\"\")"=w360) -> ("States Out"=w359:string)  [unwired: 14 in]
      }
      frame "File: Location" {
        n115 = Current VI's Path() -> (path=w369:path)
        n116 = Strip Path(path=w369) -> (stripped path=w361:path)  [unwired: 1 out]
        n117 = Build Path(base path=w361, name or relative path="Data") -> (appended path=w363:path)
        n118 = control-ref of="FileExplore"() -> (w365:refnum<vi>)
        n119 = call "Init_Open_Close.vi"("pattern"="*xls", "path to start the search"=w363, "Tree In"=w365) -> ("Tree Out"=w364:refnum<vi>)  [unwired: 6 in, 2 out]
        n120 = Bundle By Name(cluster=w367, "FilePath"=w363, "Tree Out"=w364) -> (w366:T8)
        n121 = call "Add State(s) to Queue__jki_lib_state_machine.vi"("State(s) in (\"\")"=w374) -> ("States Out"=w373:string)  [unwired: 14 in]
      }
      frame "File: ManueRead" {
        n122 = Unbundle By Name(w378) -> ("FilePath"=w376:path)
        n123 = Build Path(base path=w376, name or relative path="DWTT060916-1-Raw.txt") -> (appended path=w375:path)
        n124 = Bundle By Name(cluster=w378, "FilePath"=w375) -> (w379:T8)
        n125 = call "Add State(s) to Queue__jki_lib_state_machine.vi"("State(s) in (\"\")"=w384) -> ("States Out"=w383:string)  [unwired: 14 in]
      }
      frame "FIle: Single" {
        # "用户选中一个文件，查看图像。"
        n126 = Unbundle By Name(w386) -> ("RawData"=w389:T14, "FilePathArray"=w392:path[])
        n127 = Index Array(array=w392, index=0) -> (element=w390:path)
        n128 = call "ReadFromSIngelFile.vi"("FilePath"=w390, "RawData"=w389) -> ("XYData"=w387:cluster{"X":dbl[], "Y":dbl[]}[], "RawDataOut"=w388:T14)  [unwired: 7 in, 1 out]
        n129 = Bundle By Name(cluster=w386, "RawData"=w388, "XYData"=w387) -> (w385:T8)
        n130 = call "Add State(s) to Queue__jki_lib_state_machine.vi"("State(s) in (\"\")"=w397) -> ("States Out"=w396:string)  [unwired: 14 in]
      }
      frame "File: Multi" {
        # "用户选中多个文件，查看图像。"
        n131 = Unbundle By Name(w401) -> ("RawData"=w403:T14, "FilePathArray"=w402:path[])
        n132 = call "ReadFromMultiFile.vi"("FilePathArray"=w402, "RawData"=w403) -> ("MultiPlot"=w398:T12, "RawDataOut"=w399:T14)  [unwired: 7 in, 1 out]
        n133 = Bundle By Name(cluster=w401, "RawData"=w399, "MultiPlot"=w398) -> (w400:T8)
        n134 = call "Add State(s) to Queue__jki_lib_state_machine.vi"("State(s) in (\"\")"=w408) -> ("States Out"=w407:string)  [unwired: 14 in]
      }
      frame "---------- XYGraph ----------" {
        n135 = call "Add State(s) to Queue__jki_lib_state_machine.vi"("State(s) in (\"\")"=w414) -> ("States Out"=w413:string)  [unwired: 14 in]
      }
      frame "XY: GraphChoose" {
        # "XY: GraphChoose    --   控制图形的显示。"
        n136 = Unbundle By Name(w416) -> ("XYData"=w419:cluster{"X":dbl[], "Y":dbl[]}[], "MultiPlot"=w418:T12, "ChooseGraph"=w417:T5)
        n137 = case shown="\"MultiFile\"" w420 {
          tunnel: w419 -> [w430 _]
          tunnel: w418 -> [_ w435]
          tunnel: w417 -> [w429 w434]
          tunnel: w416 -> [w428 w433]
          tunnel: [w426 w432] -> w415
          frame "SingelFile", Default {
            n138 = call "SingleFileGraphChoose.vi"("Relationship"=w429, "XYData"=w430) -> ("XYDataOut"=w427:cluster{"X":dbl[], "Y":dbl[]}[])  [unwired: 9 in]
            n139 = Bundle By Name(cluster=w428, "XYDataResult"=w427) -> (w426:T8)
          }
          frame "MultiFile" {
            n140 = call "MultiFileGraphChoose.vi"("Relationship"=w434, "MultiPlot"=w435) -> ("XYDataOut"=w431:cluster{"X":dbl[], "Y":dbl[]}[])  [unwired: 9 in]
            n141 = Bundle By Name(cluster=w433, "XYDataResult"=w431) -> (w432:T8)
          }
        }
        n142 = call "Add State(s) to Queue__jki_lib_state_machine.vi"("State(s) in (\"\")"=w425) -> ("States Out"=w424:string)  [unwired: 14 in]
      }
      frame "XY: ChangeScaleLable" {
        # "T(ms)          \tForce(kN)\t          Des(mm)\t           V(m1s)\t             E(kJ)"
        # "修改XY图形的坐标Lable。"
        # "t_ms   \tForce_kN\t des_mm\t v_m1s\t  E_kJ"
        n143 = Unbundle By Name(w439) -> ("ScaleLabelText"=w438:cluster{"X":string, "Y":string})
        n144 = Unbundle By Name(w438) -> ("X"=w437:string, "Y"=w436:string)
        n145 = property on="MainXY" class="XYGraph (strict)"("XScale.NameLbl.Text"=w437, "YScale.NameLbl.Text"=w436) -> ()  [unwired: 2 in, 2 out]
        n146 = call "Add State(s) to Queue__jki_lib_state_machine.vi"("State(s) in (\"\")"=w444) -> ("States Out"=w443:string)  [unwired: 14 in]
      }
      frame "XY: MainUpdate" {
        n147 = Unbundle By Name(w446) -> ("XYDataResult"=→"MainXY":cluster{"X":dbl[], "Y":dbl[]}[])
        n148 = call "Add State(s) to Queue__jki_lib_state_machine.vi"("State(s) in (\"\")"=w451) -> ("States Out"=w450:string)  [unwired: 14 in]
      }
      frame "---------- New Category2 ----------" {
        n149 = call "Add State(s) to Queue__jki_lib_state_machine.vi"("State(s) in (\"\")"=w457) -> ("States Out"=w456:string)  [unwired: 14 in]
      }
      frame "New Category: 1" {
        n150 = call "Add State(s) to Queue__jki_lib_state_machine.vi"("State(s) in (\"\")"=w463) -> ("States Out"=w462:string)  [unwired: 14 in]
      }
      frame "New Category: 2" {
        n151 = call "Add State(s) to Queue__jki_lib_state_machine.vi"("State(s) in (\"\")"=w469) -> ("States Out"=w468:string)  [unwired: 14 in]
      }
    }
  }
  n152 = disable-structure shown="Disabled" {
    frame Disabled {
    }
    frame Enabled {
    }
  }
  n153 = property on="Wave Select" class="Ring (strict)"("Strings []"=string[] ["力/时间", "力/位移", "能量/位移", "位移/时间", "能量/时间", "速度/时间"]) -> ()  [unwired: 2 in, 2 out]
